vi "SPI Write and Read.vi"(8 "error in (no error)":errorcluster, 9 "Chip Select":u8, 10 "SPI Command":u64, 11 "All SPI Settings":T1={"SPI Signal Settings"={"SCLK"={"Signal"="sbRIO-9651 Socket\\PMOD1_Pin4_out", "Signal_Enable"="sbRIO-9651 Socket\\PMOD1_Pin4_enable", "Output?"=FALSE}, "Signal Settings"={"MISO"="sbRIO-9651 Socket\\PMOD1_Pin3_in", "Signal_Enable"="sbRIO-9651 Socket\\PMOD1_Pin4_enable", "Output?"=FALSE}, "MOSI"={"Signal"="sbRIO-9651 Socket\\PMOD1_Pin4_out", "Signal_Enable"="sbRIO-9651 Socket\\PMOD1_Pin4_enable", "Output?"=FALSE}, "CS0"={"Signal"="sbRIO-9651 Socket\\PMOD1_Pin4_out", "Signal_Enable"="sbRIO-9651 Socket\\PMOD1_Pin4_enable", "Output?"=FALSE}, "CS1"={"Signal"="sbRIO-9651 Socket\\PMOD1_Pin4_out", "Signal_Enable"="sbRIO-9651 Socket\\PMOD1_Pin4_enable", "Output?"=FALSE}, "CS2"={"Signal"="sbRIO-9651 Socket\\PMOD1_Pin4_out", "Signal_Enable"="sbRIO-9651 Socket\\PMOD1_Pin4_enable", "Output?"=FALSE}, "CS3"={"Signal"="sbRIO-9651 Socket\\PMOD1_Pin4_out", "Signal_Enable"="sbRIO-9651 Socket\\PMOD1_Pin4_enable", "Output?"=FALSE}, "CS4"={"Signal"="sbRIO-9651 Socket\\PMOD1_Pin4_out", "Signal_Enable"="sbRIO-9651 Socket\\PMOD1_Pin4_enable", "Output?"=FALSE}, "CS5"={"Signal"="sbRIO-9651 Socket\\PMOD1_Pin4_out", "Signal_Enable"="sbRIO-9651 Socket\\PMOD1_Pin4_enable", "Output?"=FALSE}}, "SPI Internal Signals"={"DLU To SPI Engine Data FIFO"="DLU To SPI Engine Data", "SPI Engine to DLU Data FIFO"="SPI Engine to DLU Data", "Data to SPI Engine (Cache) Register"="Data to SPI Engine (Cache)", "SPI PHY Settings to SPI Engine (Cahche) Register"="SPI PHY Settings to SPI Engine (Cache)"}, "SPI PHY Settings"={"Divide Value"=0, "Transfer Length (bits)"=0, "CS Asserted Polarity"=FALSE, "Clock Polarity (CPOL)"=FALSE, "Clock Phase (CPHA)"=FALSE, "Lengthen MISO Setup"=FALSE, "Direction Change Bit"=0, "MOSI Starts as Output"=FALSE, "Tristatable MOSI"=FALSE}, "SPI Engine Source"="120MHz"} {"SPI PHY Settings"."Direction Change Bit" max=64 step=1; "SPI PHY Settings"."Transfer Length (bits)" min=1 max=64 step=1}) -> (0 "error out":errorcluster, 1 "Read Attempts":i32, 2 "SPI Return Data":u64, 3 "Dup All SPI Settings":T1={"SPI Signal Settings"={"SCLK"={"Signal"="sbRIO-9651 Socket\\PMOD1_Pin4_out", "Signal_Enable"="sbRIO-9651 Socket\\PMOD1_Pin4_enable", "Output?"=FALSE}, "Signal Settings"={"MISO"="sbRIO-9651 Socket\\PMOD1_Pin3_in", "Signal_Enable"="sbRIO-9651 Socket\\PMOD1_Pin4_enable", "Output?"=FALSE}, "MOSI"={"Signal"="sbRIO-9651 Socket\\PMOD1_Pin4_out", "Signal_Enable"="sbRIO-9651 Socket\\PMOD1_Pin4_enable", "Output?"=FALSE}, "CS0"={"Signal"="sbRIO-9651 Socket\\PMOD1_Pin4_out", "Signal_Enable"="sbRIO-9651 Socket\\PMOD1_Pin4_enable", "Output?"=FALSE}, "CS1"={"Signal"="sbRIO-9651 Socket\\PMOD1_Pin4_out", "Signal_Enable"="sbRIO-9651 Socket\\PMOD1_Pin4_enable", "Output?"=FALSE}, "CS2"={"Signal"="sbRIO-9651 Socket\\PMOD1_Pin4_out", "Signal_Enable"="sbRIO-9651 Socket\\PMOD1_Pin4_enable", "Output?"=FALSE}, "CS3"={"Signal"="sbRIO-9651 Socket\\PMOD1_Pin4_out", "Signal_Enable"="sbRIO-9651 Socket\\PMOD1_Pin4_enable", "Output?"=FALSE}, "CS4"={"Signal"="sbRIO-9651 Socket\\PMOD1_Pin4_out", "Signal_Enable"="sbRIO-9651 Socket\\PMOD1_Pin4_enable", "Output?"=FALSE}, "CS5"={"Signal"="sbRIO-9651 Socket\\PMOD1_Pin4_out", "Signal_Enable"="sbRIO-9651 Socket\\PMOD1_Pin4_enable", "Output?"=FALSE}}, "SPI Internal Signals"={"DLU To SPI Engine Data FIFO"="DLU To SPI Engine Data", "SPI Engine to DLU Data FIFO"="SPI Engine to DLU Data", "Data to SPI Engine (Cache) Register"="Data to SPI Engine (Cache)", "SPI PHY Settings to SPI Engine (Cahche) Register"="SPI PHY Settings to SPI Engine (Cache)"}, "SPI PHY Settings"={"Divide Value"=0, "Transfer Length (bits)"=0, "CS Asserted Polarity"=FALSE, "Clock Polarity (CPOL)"=FALSE, "Clock Phase (CPHA)"=FALSE, "Lengthen MISO Setup"=FALSE, "Direction Change Bit"=0, "MOSI Starts as Output"=FALSE, "Tristatable MOSI"=FALSE}, "SPI Engine Source"="120MHz"} {"SPI PHY Settings"."Direction Change Bit" max=64 step=1; "SPI PHY Settings"."Transfer Length (bits)" min=1 max=64 step=1})   [LabVIEW 2014]
uses:
  Controls/All SPI Settings.ctl
  Controls/SPI Settings.ctl
  Controls/Signal Properties.ctl
  Controls/Internal Data (SPI API).ctl
  <userlib>/_NI SPI IP/FPGA/Controllers/Public/Transfer Settings.ctl
  <vilib>/Platform/TimedLoop/XDataNode/timing_clust.ctl
  <vilib>/Platform/TimedLoop/XDataNode/nitl_modes.ctl
  <vilib>/Platform/TimedLoop/XDataNode/wakeup.ctl
  <vilib>/rvi/Emulation/niFpgaGetClockAttributes.vi
  <vilib>/rvi/Emulation/niFpgaSctlEmulationGetInTimedLoop.vi
  <vilib>/rvi/Emulation/niFpgaEmulationReportErrorSimple.vi
  <vilib>/rvi/Emulation/niFpgaCriticalErrorInLSC.vi
  <vilib>/Platform/TimedLoop/XDataNode/XDataNode.xnode
  <vilib>/Platform/TimedLoop/XDataNode/XDNodeRunTimeDep.lvlib
  <userlib>/_NI SPI IP/FPGA/Controllers/NI SPI IP FPGA.lvlib
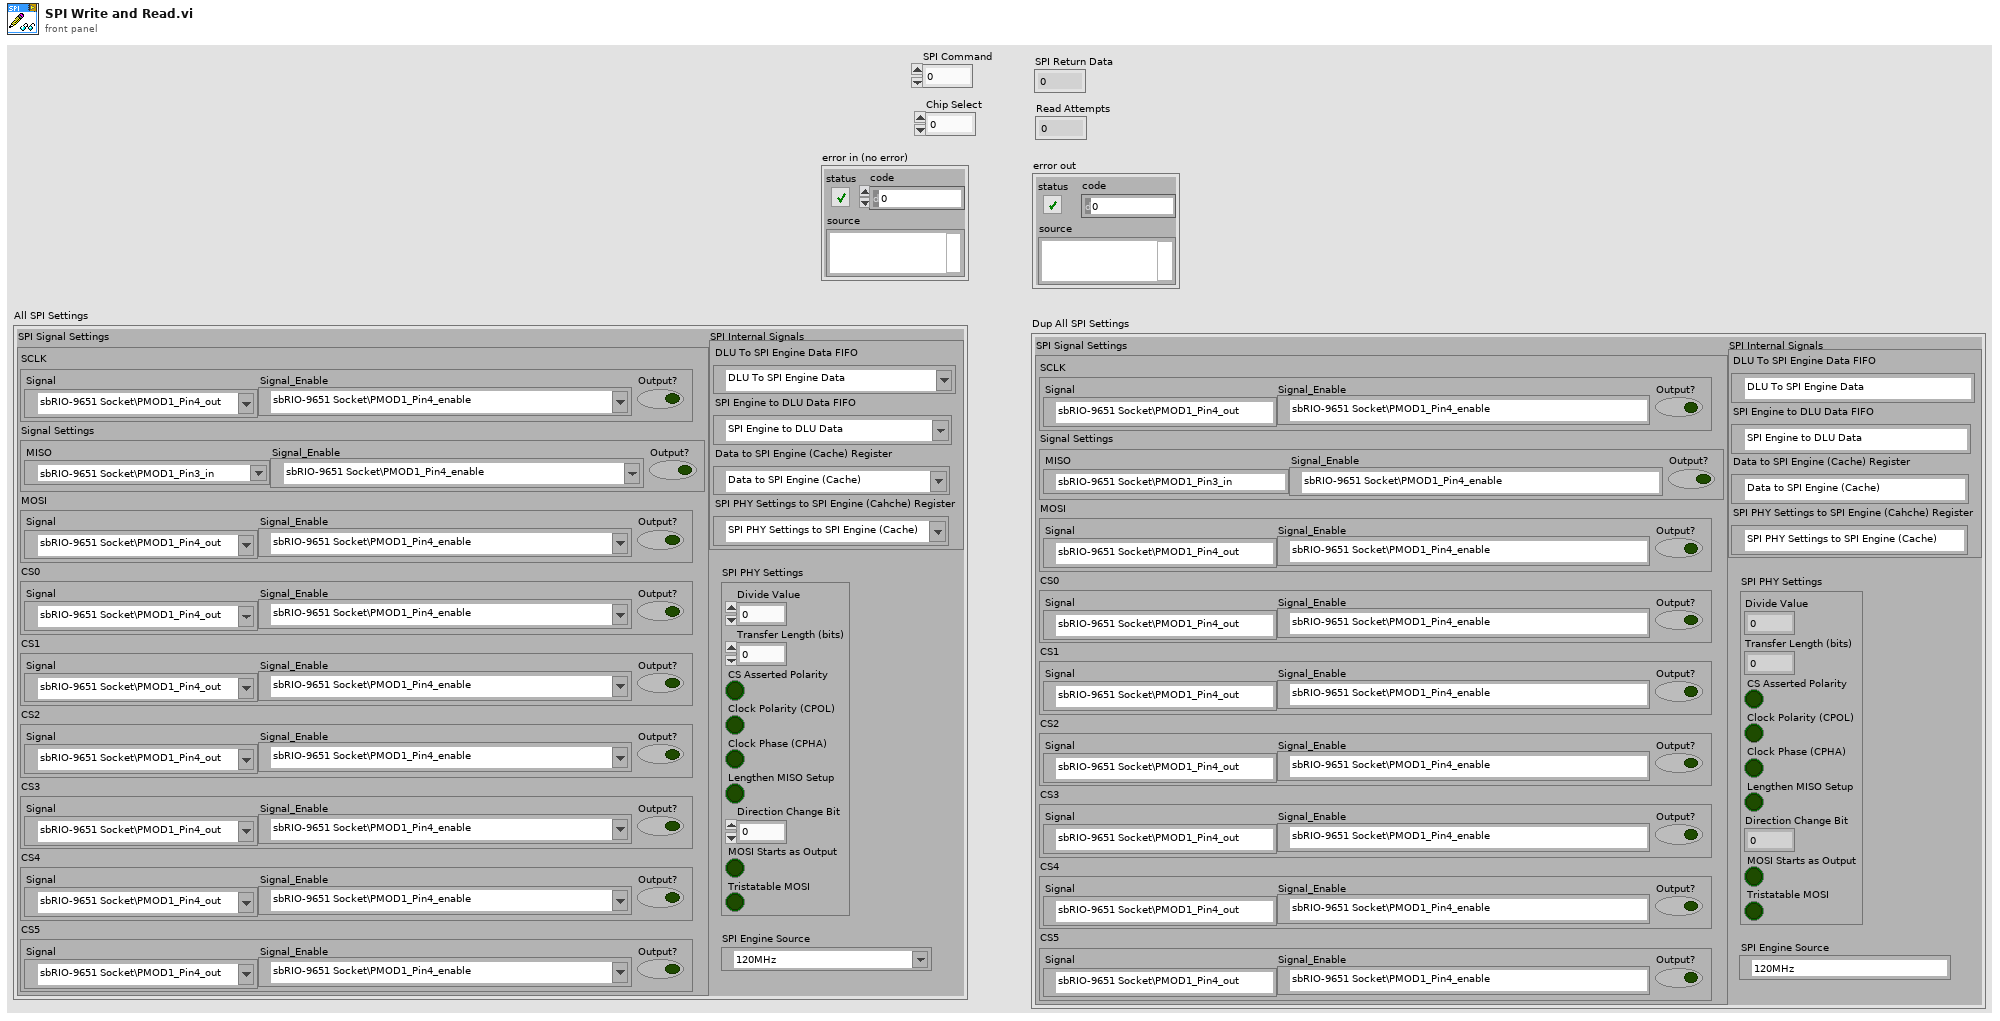
[diagram p1: front panel]
types:
  T1 = typedef "All SPI Settings.ctl" = cluster{"SPI Signal Settings":T2, "SPI Internal Signals":T4, "SPI PHY Settings":T5, "SPI Engine Source":refnum<k21>}
  T2 = typedef "SPI Settings.ctl" = cluster{"SCLK":T3, "Signal Settings":cluster{"MISO":refnum<k21>, "Signal_Enable":refnum<k21>, "Output?":bool}, "MOSI":T3, "CS0":T3, "CS1":T3, "CS2":T3, "CS3":T3, "CS4":T3, "CS5":T3}
  T3 = typedef "Signal Properties.ctl" = cluster{"Signal":refnum<k21>, "Signal_Enable":refnum<k21>, "Output?":bool}
  T4 = typedef "Internal Data (SPI API).ctl" = cluster{"DLU To SPI Engine Data FIFO":refnum<k21>, "SPI Engine to DLU Data FIFO":refnum<k21>, "Data to SPI Engine (Cache) Register":refnum<k21>, "SPI PHY Settings to SPI Engine (Cahche) Register":refnum<k21>}
  T5 = typedef "NI SPI IP FPGA.lvlib/Transfer Settings.ctl" = cluster{"Divide Value":u8, "Transfer Length (bits)":u8, "CS Asserted Polarity":bool, "Clock Polarity (CPOL)":bool, "Clock Phase (CPHA)":bool, "Lengthen MISO Setup":bool, "Direction Change Bit":u8, "MOSI Starts as Output":bool, "Tristatable MOSI":bool}
  T6 = typedef "XDNodeRunTimeDep.lvlib/timing_clust.ctl" = cluster{"Expected End [f-1]":u64, "Actual End [f-1]":u64, "Finished Late? [f-1]":bool, "Expected End [i-1]":u64, "Actual End [i-1]":u64, "Finished Late? [i-1]":bool, "Expected Start [i]":u64, "Actual Start [i]":u64, "Expected Start [f]":u64, "Actual Start [f]":u64, "Source Name":string, "Structure Name":string, "Period":i64, "Deadline":i64, "Offset":i64, "Start":i64, "Priority":i32, "Timeout":i32, "Mode":T7, "Wakeup Reason":T8, "Error":errorcluster, "Source Type":string, "Secondary Source Type":string, "Global End Time":u64, "Global Start Time":u64, "Frame Duration":u64, "Iteration Duration":u64, "Assigned CPU":i32, "I/O Scan Engine Mode":u32}
  T7 = typedef "XDNodeRunTimeDep.lvlib/nitl_modes.ctl" = enum32{"No Change", "Process missed periods, maintain original phase", "Discard missed periods, maintain original phase", "Process missed periods, ignore original phase", "Discard missed periods, ignore original phase"}
  T8 = typedef "XDNodeRunTimeDep.lvlib/wakeup.ctl" = enum32{"Normal", "Aborted", "Asynchronous wakeup", "Timing source error", "Timed loop error", "Timeout"}
  T9 = typedef "SPI Response Information.ctl" = cluster{"Data to Node":u64, "Node Id":u16}
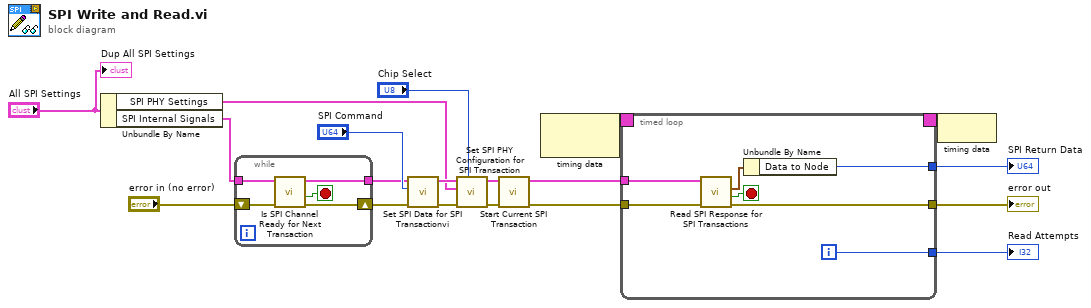
[diagram p0: block diagram]
diagram:
  n1 = Unbundle By Name("All SPI Settings") -> ("SPI PHY Settings"=w1:T5, "SPI Internal Signals"=w2:T4)
  n2 = while {
    shift-right: [w24] -> w4
    shift-left: "error in (no error)" -> [w21]
    tunnel: w2 -> [w22]
    tunnel: [w23] -> w5
    stop <- w20 stop-if-true
    n3 = call "Is SPI Channel Ready for Next Transaction.vi"("error in"=w21, "Private Data In"=w22) -> ("error out"=w24:errorcluster, "SPI Channel Ready"=w20:bool, "Private Data Out"=w23:T4)  [unwired: 6 in, 1 out]
  }
  n4 = call "Set SPI Data for SPI Transactionvi.vi"("error in"=w4, "Data In"="SPI Command", "Private Data In"=w5) -> ("error out"=w11:errorcluster, "Private Data Out"=w10:T4)  [unwired: 7 in]
  n5 = call "Set SPI PHY Configuration for SPI Transaction.vi"("Chip Select"="Chip Select", "error in"=w11, "SPI PHY Settings"=w1, "Private Data In"=w10) -> ("error out"=w14:errorcluster, "Private Data Out"=w13:T4)  [unwired: 6 in]
  n6 = call "Start Current SPI Transaction.vi"("error in"=w14, "Private Data In"=w13) -> ("error out"=w9:errorcluster, "Private Data Out"=w15:T4)  [unwired: 7 in, 1 out]
  n7 = node-c288() -> (w19:T6)  [unwired: 1 in]
  n8 = timed-loop {
    timing: w19 -> [_]
    timing-out: [_] -> w18
    tunnel: w9 -> [w31]
    tunnel: w15 -> [w30]
    tunnel: [w26] -> w8
    tunnel: [w27] -> w7
    tunnel: [w25] -> w17
    i -> [w25]
    stop <- w29 stop-if-true
    n9 = call "Read SPI Response for SPI Transactions.vi"("error in"=w31, "Private Data In"=w30) -> ("error out"=w27:errorcluster, "Read Data Valid?"=w29:bool, "Read Data"=w28:T9)  [unwired: 6 in, 1 out]
    n10 = Unbundle By Name(w28) -> ("Data to Node"=w26:u64)
  }
  "Read Attempts" <- w17
  "SPI Return Data" <- w8
  "error out" <- w7
  n11 = node-c288(w18) -> ()
  "Dup All SPI Settings" <- "All SPI Settings"
